vi "Calculator.vi"(7 "Operator":T1(ring), 8 "error in (no error)":errorcluster, 10 "y":dbl, 11 "x":dbl) -> (0 "error out":errorcluster, 3 "Answer":dbl)   [LabVIEW 2014]
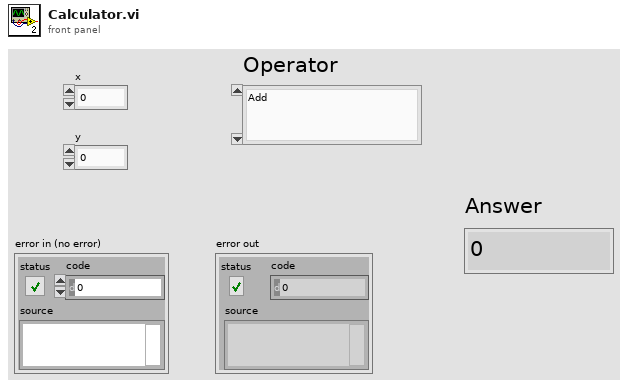
[diagram p1: front panel]
types:
  T1 = enum16{"Add", "Subtract", "Divide", "Multiply", "Power y^x"}
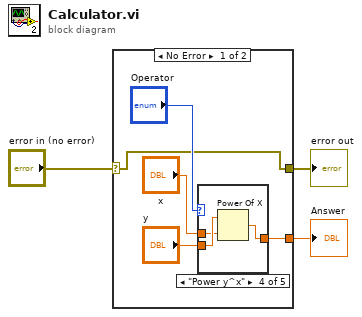
[diagram p0: block diagram]
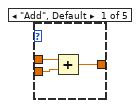
[diagram p2: hidden frame]
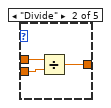
[diagram p3: hidden frame]
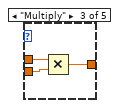
[diagram p4: hidden frame]
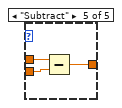
[diagram p5: hidden frame]
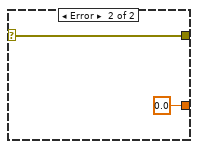
[diagram p6: hidden frame]
diagram:
  n1 = case shown="No Error" "error in (no error)" {
    selector: "error in (no error)" -> [w4 w24]
    tunnel: [w5 0.0] -> w3
    tunnel: [w4 w24] -> w1
    frame No Error {
      n2 = case shown="\"Power y^x\"" "Operator" {
        tunnel: "x" -> [w11 w14 w17 w19 w23]
        tunnel: "y" -> [w10 w13 w16 w20 w22]
        tunnel: [w9 w12 w15 w18 w21] -> w5
        frame "Add", Default {
          n3 = Add(x=w11, y=w10) -> (x+y=w9:dbl)
        }
        frame "Divide" {
          n4 = Divide(x=w14, y=w13) -> (x/y=w12:dbl)
        }
        frame "Multiply" {
          n5 = Multiply(x=w17, y=w16) -> (x*y=w15:dbl)
        }
        frame "Power y^x" {
          n6 = Power Of X(1:w19, 2:w20) -> (0:w18:dbl)
        }
        frame "Subtract" {
          n7 = Subtract(x=w23, y=w22) -> (x-y=w21:dbl)
        }
      }
    }
    frame Error {
    }
  }
  "Answer" <- w3
  "error out" <- w1
